vi "Initialize Hardware.vi"(8 "error in (no error)":errorcluster, 9 "Session Setting":T1={"cluster (:memory:)"=":memory:", "interface"=""}, 10 "DAQ Type":enum16{"Hardware", "Simulation"}(ring), 11 "PXI 8513 in":refnum<class "PXI 8513.lvclass">) -> (0 "error out":errorcluster, 3 "PXI 8513 out":refnum<class "PXI 8513.lvclass">)   [LabVIEW 2023, in "CAN.lvlib" / "PXI 8513.lvclass"]
uses:
  PXI 8513.lvclass
  PXI 8513.lvclass/PXI 8513.ctl
  <vilib>/xnet/xnet.llb/XNET Create Session (Frame Output Stream).vi
panel:
  in  "Connection Ref":variant
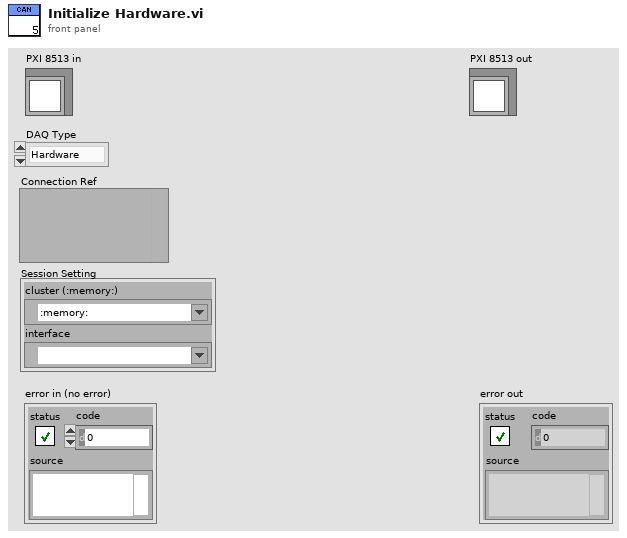
[diagram p1: front panel]
types:
  T1 = cluster{"cluster (:memory:)":refnum<k21>, "interface":refnum<k21>}
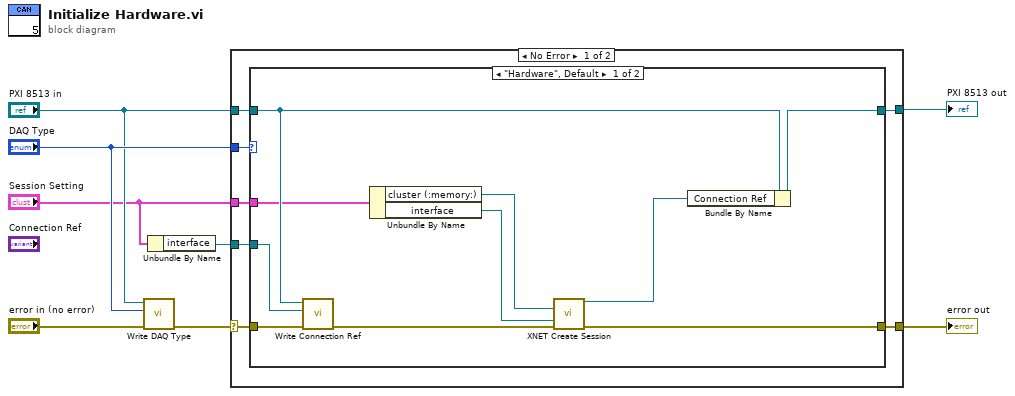
[diagram p0: block diagram]
diagram:
  n1 = call-dynamic "Write DAQ Type.vi"("error in (no error)"="error in (no error)", "DAQ Type"="DAQ Type", "PXI 8513 in"="PXI 8513 in") -> ("error out"=w7:errorcluster)  [unwired: 7 in, 1 out]
  n2 = Unbundle By Name("Session Setting") -> ("interface"=w1:refnum<k21>)
  n3 = case shown="No Error" w7 {
    selector: w7 -> [w15 w28]
    tunnel: "DAQ Type" -> [w14 _]
    tunnel: w1 -> [w13 _]
    tunnel: "PXI 8513 in" -> [w12 w29]
    tunnel: [w11 w29] -> w4
    tunnel: "Session Setting" -> [w10 _]
    tunnel: [w9 w28] -> w3
    frame No Error {
      n4 = case shown="\"Hardware\", Default" w14 {
        tunnel: w15 -> [w25 w26]
        tunnel: w13 -> [w24 _]
        tunnel: w12 -> [w23 w27]
        tunnel: [w18 w27] -> w11
        tunnel: w10 -> [w19 _]
        tunnel: [w16 w26] -> w9
        frame "Hardware", Default {
          n5 = call-dynamic "Write Connection Ref.vi"("error in (no error)"=w25, "Connection Ref"=w24, "PXI 8513 in"=w23) -> ("error out"=w22:errorcluster)  [unwired: 7 in, 1 out]
          n6 = Unbundle By Name(w19) -> ("cluster (:memory:)"=w20:refnum<k21>, "interface"=w21:refnum<k21>)
          n7 = call-poly <vilib>:"XNET Create Session.vi"("cluster (:memory:)"=w20, "interface"=w21, "error in (no error)"=w22) -> ("session out"=w17:refnum<k21>, "error out"=w16:errorcluster)  [unwired: 11 in]
          n8 = Bundle By Name(cluster=w23, "Connection Ref"=w17) -> (w18:refnum<class "PXI 8513.lvclass">)
        }
        frame "Simulation" {
        }
      }
    }
    frame Error {
    }
  }
  "error out" <- w3
  "PXI 8513 out" <- w4
